vi "AttributesInfo.vi"() -> ()   [LabVIEW 2013, in "examples.lvlib"]
uses:
  examples.lvlib
  vis/lv-2013/tango_vi.llb/tango.lvlib
panel:
  out "attributes_info":T1(array[cluster])
  in  "device name":string="sys/tg_test/1"
  out "success":bool
  # "AttributeInfo.r/w access\n-----------------------\n\tREAD = 0\n READ_WITH_WRITE = 1\n WRITE = 2\n READ_WRITE = 3"
  # "AttributeInfo.data-type\n-----------------------\n\tDEV_VOID = 0\n\tDEV_BOOLEAN = 1\n\tDEV_SHORT = 2\n\tDEV_LONG = 3\n\tDEV_FLOAT = 4\n\tDEV_DOUBLE = 5\n\tDEV_USHORT = 6\n\tDEV_ULONG = 7\n\tDEV_STRING = 8\n\tDEVVAR_CHARARRAY = 9\n\tDEVVAR_SHORTARRAY = 10\n\tDEVVAR_LONGARRAY = 11\n\tDEVVAR_FLOATARRAY = 12\n\tDEVVAR_DOUBLEARRAY = 13\n\tDEVVAR_USHORTARRAY = 14\n\tDEVVAR_ULONGARRAY = 15\n\tDEVVAR_STRINGARRAY = 16\n\tDEVVAR_LONGSTRINGARRAY = 17\n\tDEVVAR_DOUBLESTRINGARRAY = 18\n\tDEV_STATE = 19\n\tCONST_DEV_STRING = 20\n\tDEVVAR_BOOLEANARRAY = 21\n\tDEV_UCHAR = 22\n\tDEV_LONG64 = 23\n\tDEV_ULONG64 = 24\n\tDEVVAR_LONG64ARRAY = 25\n\tDEVVAR_ULONG64ARRAY = 26\n\tDEV_INT = 27\n\tDEV_ENCODED = 28"
  # "AttributeInfo.format\n-----------------------\n\tSCALAR = 0\n SPECTRUM = 1\n IMAGE = 2"
  # "AttributeInfo.level\n-----------------------\n\tOPERATOR = 0\n EXPERT = 1"
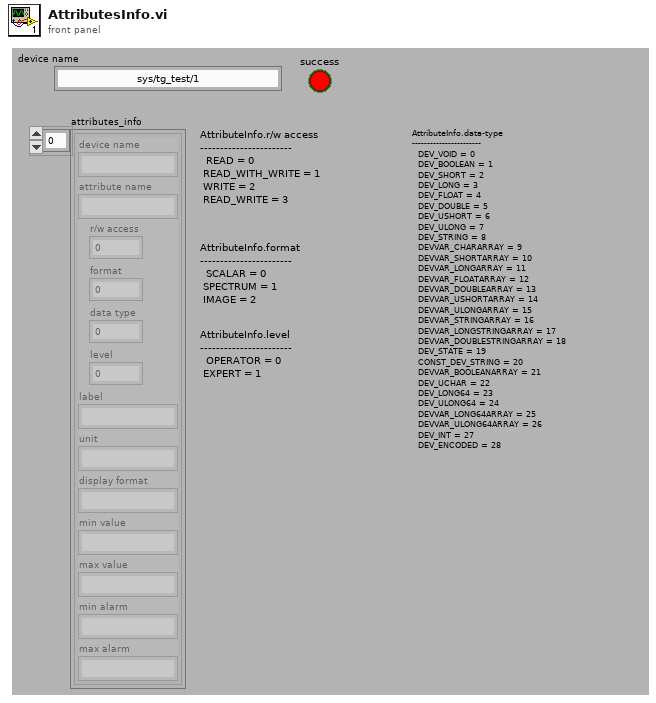
[diagram p1: front panel]
types:
  T1 = cluster{"device name":string, "attribute name":string, "r/w access":i16, "format":i16, "data type":i16, "level":i16, "label":string, "unit":string, "display format":string, "min value":string, "max value":string, "min alarm":string, "max alarm":string}[]
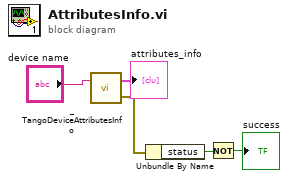
[diagram p0: block diagram]
diagram:
  n1 = call "_TangoDeviceAttributesInfo.vi"("device name"="device name") -> ("error out"=w4:errorcluster, "attributes_info"=→"attributes_info":T1)  [unwired: 1 in]
  n2 = Unbundle By Name(w4) -> ("status"=w3:bool)
  n3 = Not(x=w3) -> (.not. x?=→"success":bool)
